vi "Write conn.vi"(8 "error in (no error)":errorcluster, 10 "conn":refnum<vi>, 11 "instrXX in":refnum<class "instrXX.lvclass">) -> (0 "error out":errorcluster, 3 "instrXX out":refnum<class "instrXX.lvclass">)   [LabVIEW 2017, in "instrXX.lvclass"]
uses:
  instrXX.lvclass
  instrXX.lvclass/instrXX.ctl
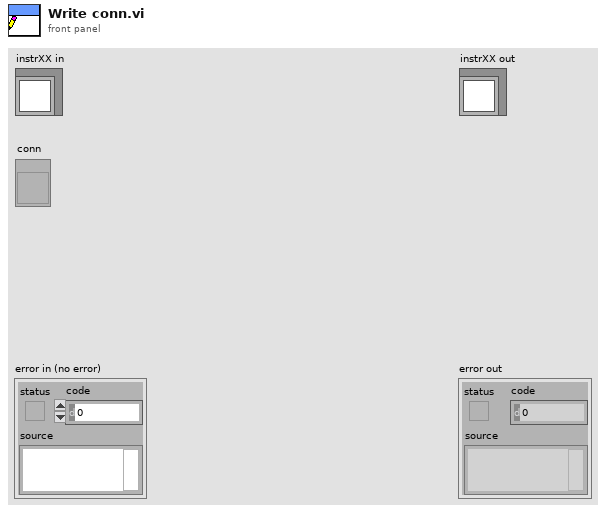
[diagram p1: front panel]
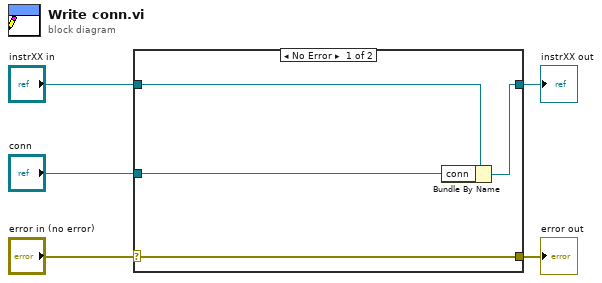
[diagram p0: block diagram]
diagram:
  n1 = case shown="No Error" "error in (no error)" {
    selector: "error in (no error)" -> [w9 w10]
    tunnel: [w9 w10] -> w4
    tunnel: [w7 w11] -> w2
    tunnel: "instrXX in" -> [w8 w11]
    tunnel: "conn" -> [w6 _]
    frame No Error {
      n2 = Bundle By Name(cluster=w8, "conn"=w6) -> (w7:refnum<class "instrXX.lvclass">)
    }
    frame Error {
    }
  }
  "error out" <- w4
  "instrXX out" <- w2
